vi "ScanFrontEnd.vi"(8 "error in (no error)":errorcluster, 11 "Scan Action":i32) -> (0 "error out":errorcluster, 3 "Scan Error":errorcluster)   [LabVIEW 2011]
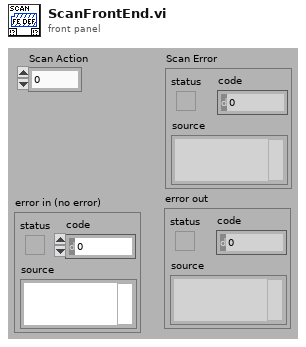
[diagram p1: front panel]
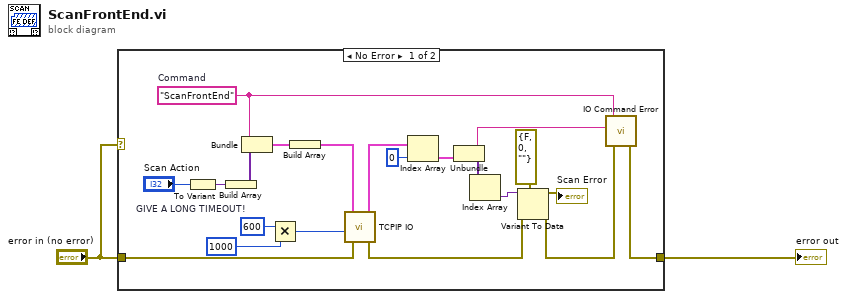
[diagram p0: block diagram]
diagram:
  n1 = case shown="No Error" "error in (no error)" {
    tunnel: "error in (no error)" -> [w19 w24]
    tunnel: [w16 w24] -> w2
    frame No Error {
      w5 = 600  # GIVE A LONG TIMEOUT!
      w15 = "ScanFrontEnd"  # Command
      n2 = To Variant(anything="Scan Action") -> (Variant=w20:variant)
      n3 = Build Array(w20) -> (w23:variant[])
      n4 = Bundle("Command"=w15, w23) -> (w22:cluster{"Command":string, variant[]})  [unwired: 1 out]
      n5 = Multiply(x=w5, y=1000 ("Semaphore TMO\n(10000 ms)")) -> (x*y=w6:i32)
      n6 = Build Array(w22) -> (w14:cluster{"Command":string, variant[]}[])
      n7 = call "TCPIP IO.vi"("error in (no error)"=w19, "TCP TMO\n(10000 ms)"=w6, "Commands"=w14) -> ("error out"=w18:errorcluster, "Responses"=w13:cluster{string, variant[]}[])  [unwired: 1 in, 2 out]
      n8 = Index Array(array=w13, index=0) -> (element=w12:cluster{string, variant[]})
      n9 = Unbundle(w12) -> (w11:string, w10:variant[])
      n10 = Index Array(array=w10) -> (element=w9:variant)  [unwired: 1 in]
      n11 = Variant To Data(error in=w18, type=errorcluster {"status"=FALSE, "code"=0, "source"=""}, Variant=w9) -> (data=→"Scan Error":errorcluster, error out=w17:errorcluster)
      n12 = call "IO Command Error.vi"("error in (no error)"=w17, "Command Returned (\"\")"=w11, "Command Sent (\"\")"=w15) -> ("error out"=w16:errorcluster)  [unwired: 4 out]
    }
    frame Error {
    }
  }
  "error out" <- w2
